vi "select_initial_all.vi"(10 "Column table":string[](array[string]), 11 "table":string) -> (2 "Data to write":bool, 3 "parameters":string)   [LabVIEW 2019, in "PostgreSQL.lvlib"]
uses:
  PostgreSQL.lvlib
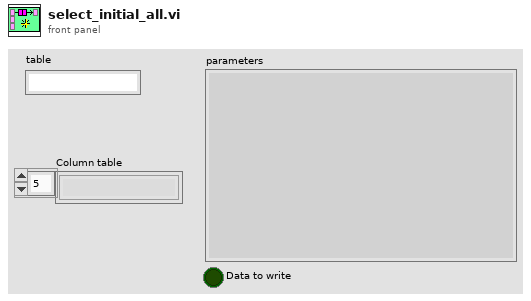
[diagram p1: front panel]
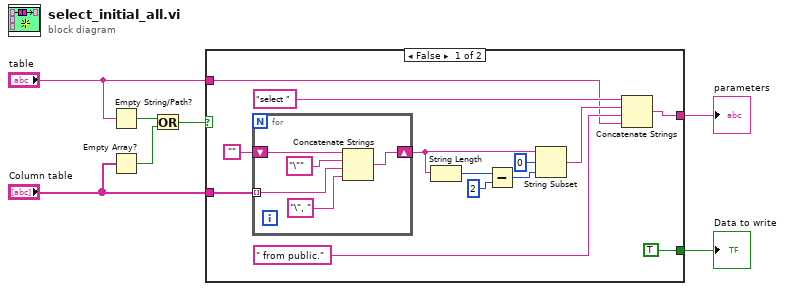
[diagram p0: block diagram]
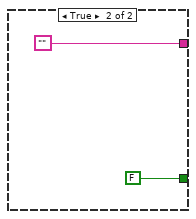
[diagram p2: hidden frame]
diagram:
  n1 = Empty String/Path?(string/path="table") -> (empty?=w4:bool)
  n2 = Empty Array?(array="Column table") -> (empty?=w3:bool)
  n3 = Or(x=w4, y=w3) -> (x .or. y?=w2:bool)
  n4 = case shown="False" w2 {
    tunnel: [w11 ""] -> w7
    tunnel: "table" -> [w10 _]
    tunnel: "Column table" -> [w9 _]
    tunnel: [TRUE FALSE] -> w1
    frame False {
      n5 = for {
        shift-right: [w23] -> w19
        shift-left: "" -> [w21]
        tunnel: w9 -> [w22] mode=indexing
        n6 = Concatenate Strings(w21, "\"" ("table"), w22, "\", " ("table")) -> (w23:string)
      }
      n7 = String Length(string=w19) -> (length=w18:i32)
      n8 = Subtract(x=w18, y=2) -> (x-y=w14:i32)
      n9 = String Subset(string=w19, offset (0)=0, length (rest)=w14) -> (substring=w16:string)
      n10 = Concatenate Strings("select " ("table"), w16, " from public." ("table"), w10) -> (w11:string)
    }
    frame True {
    }
  }
  "parameters" <- w7
  "Data to write" <- w1
